vi "WindTunnel.vi"() -> ()   [LabVIEW 2019]
uses:
  <vilib>/platform/TimedLoop/XDataNode/XDataNode.xnode
  <vilib>/Platform/TimedLoop/XDataNode/nitl_modes.ctl
  <vilib>/Platform/TimedLoop/XDataNode/XDNodeRunTimeDep.lvlib
  <vilib>/Platform/TimedLoop/XDataNode/wakeup.ctl
  <vilib>/Platform/TimedLoop/XDataNode/timing_clust.ctl
  <resource>/objmgr/ni.dex.rc
panel:
  out "save_counter":dbl
  out "saving_now":bool
  out "save_array":dbl[][](array[numeric])
  out "Aux Pressure":dbl
  out "Pitot Pressure":dbl
  out "save_file":path
  out "file_header":string[](array[string])=["%Atmospheric Pressure [Pa]", "Atmospheric Temperature [K]", "Atmospheric Density [kg/m^3]", "Airspeed [m/s]", "Pitot Dynamic Pressure [Pa]", "Aux Dynamic Pressure [Pa]", "Scanivalve Pressure 1 [Pa]", "Scanivalve Pressure 2 [Pa]", "Scanivalve Pressure 3 [Pa]", "Scanivalve Pressure 4 [Pa]", "Scanivalve Pressure 5 [Pa]", "Scanivalve Pressure 6 [Pa]", "Scanivalve Pressure 7 [Pa]", "Scanivalve Pressure 8 [Pa]", "Scanivalve Pressure 9 [Pa]", "Scanivalve Pressure 10 [Pa]", "Scanivalve Pressure 11 [Pa]", "Scanivalve Pressure 12 [Pa]", "Scanivalve Pressure 13 [Pa]", "Scanivalve Pressure 14 [Pa]", "Scanivalve Pressure 15 [Pa]", "Scanivalve Pressure 16 [Pa]", "Angle of Attack [deg]", "Sting Normal Force [N]", "Sting Axial Force [N]", "Sting Pitching Moment [Nm]", "ELD Probe X axis [mm]", "ELD Probe Y axis [mm]"]
  in  "Voltage Control":bool
  out "Connected\n 2":bool
  out "error out 2":errorcluster
  in  "stop 2":bool
  out "Connected":bool
  out "error out":errorcluster
  in  "Samples per Set to Save(Set before running)":dbl=20.0 caption="Samples per Set to Save" min=1.0 max=500.0 step=1.0 format="%#_13g"
  out "Control Voltage [V]":dbl=3.233886157886598
  out "Last Y Position Sent":dbl=336.2689146979012 format="%0.2f"
  out "Last X Position Sent":dbl=535.0482220636093 format="%0.2f"
  out "Sample Sets Sent to File":dbl=4.0
  out "Sampling Rate":dbl=500.0
  out "Airspeed Dynamic\n+/- 70 Pa {6895 Pa max}":dbl=106.03006103917599
  in  "stop":bool
  in  "Zero ELD Probe Location":bool
  in  "Desired Airspeed (m/s)":dbl(knob) min=0.0 max=40.0 step=0.01 scale=0.0..40.0 scale format="%.2g"
  out "Y":dbl=336.2689146979012 format="%.2f"
  out "X":dbl=535.0482220636093 format="%.2f"
  in  "Send Samples To File":bool
  out "Actual Airspeed [m/s]":dbl(knob) caption="m/s" scale=0.0..64.8 scale format="%_3g"
  in  "Tab Control":enum32{"Pressures", "Forces", "Angle of Attack"}(tab)
  out "Scanivalve Pressures":cluster{i32[], "Array":dbl[]}(graph)={[1, 2, 3, 4, 5, 6, 7, 8, 9, 10, 11, 12, 13, 14, 15, 16], "Array"=[107.2386417388916, 109.67449417114258, 112.26835975646972, 113.32290878295899, 113.25851020812988, 110.12275047302246, 110.01677665710449, 110.23803977966308, 111.38681907653809, 112.57089157104492, 115.55567054748535, 109.39623069763184, 115.34736213684081, 113.26969871520996, 112.33615150451661, 111.57799453735352]}
  out "Atm Density [kg/m^3]":dbl=0.9456665967088438 format="%.2g"
  out "Atm Pressure [Pa]":dbl=81675.50593656283 format="%.2f"
  out "Atm Temperature [K]":dbl=300.88201803705715 format="%.2g"
  in  "Zero Airspeed & Pressures":bool
  out "Pressures Chart":dynamicdata(graph)
  out "Forces Chart":dynamicdata(graph)
  in  "Zero Forces and Moment":bool
  out "Normal Force (N) {111.2 N max}":dbl=-0.11861150697340539 format="%#_5g"
  out "Axial Force (N) {44.5 N max}":dbl=0.06610776257324563 format="%#_5g"
  out "Pitching Moment (Nm) {5.6 Nm max}":dbl=-0.0053004445096350794 format="%#_5g"
  in  "AoA Switch":bool caption="Boolean"
  in  "Zero Angle":bool
  out "Angle of Attack Chart":dbl(graph)
  out "Angle of \nAttack":dbl=-0.004685357123962319 caption="deg ±20 Max" format="%.3g"
  # "AIRSPEED"
  # "ELD PRESSURE PROBE"
  # "SAMPLES"
  # "ELD Probe Location"
  # "mm"
  # "mm"
  # "Pa"
  # "Control Parameters:"
  # "Display Parameters:"
  # "Sting Balance Reading"
  # "Manual Input"
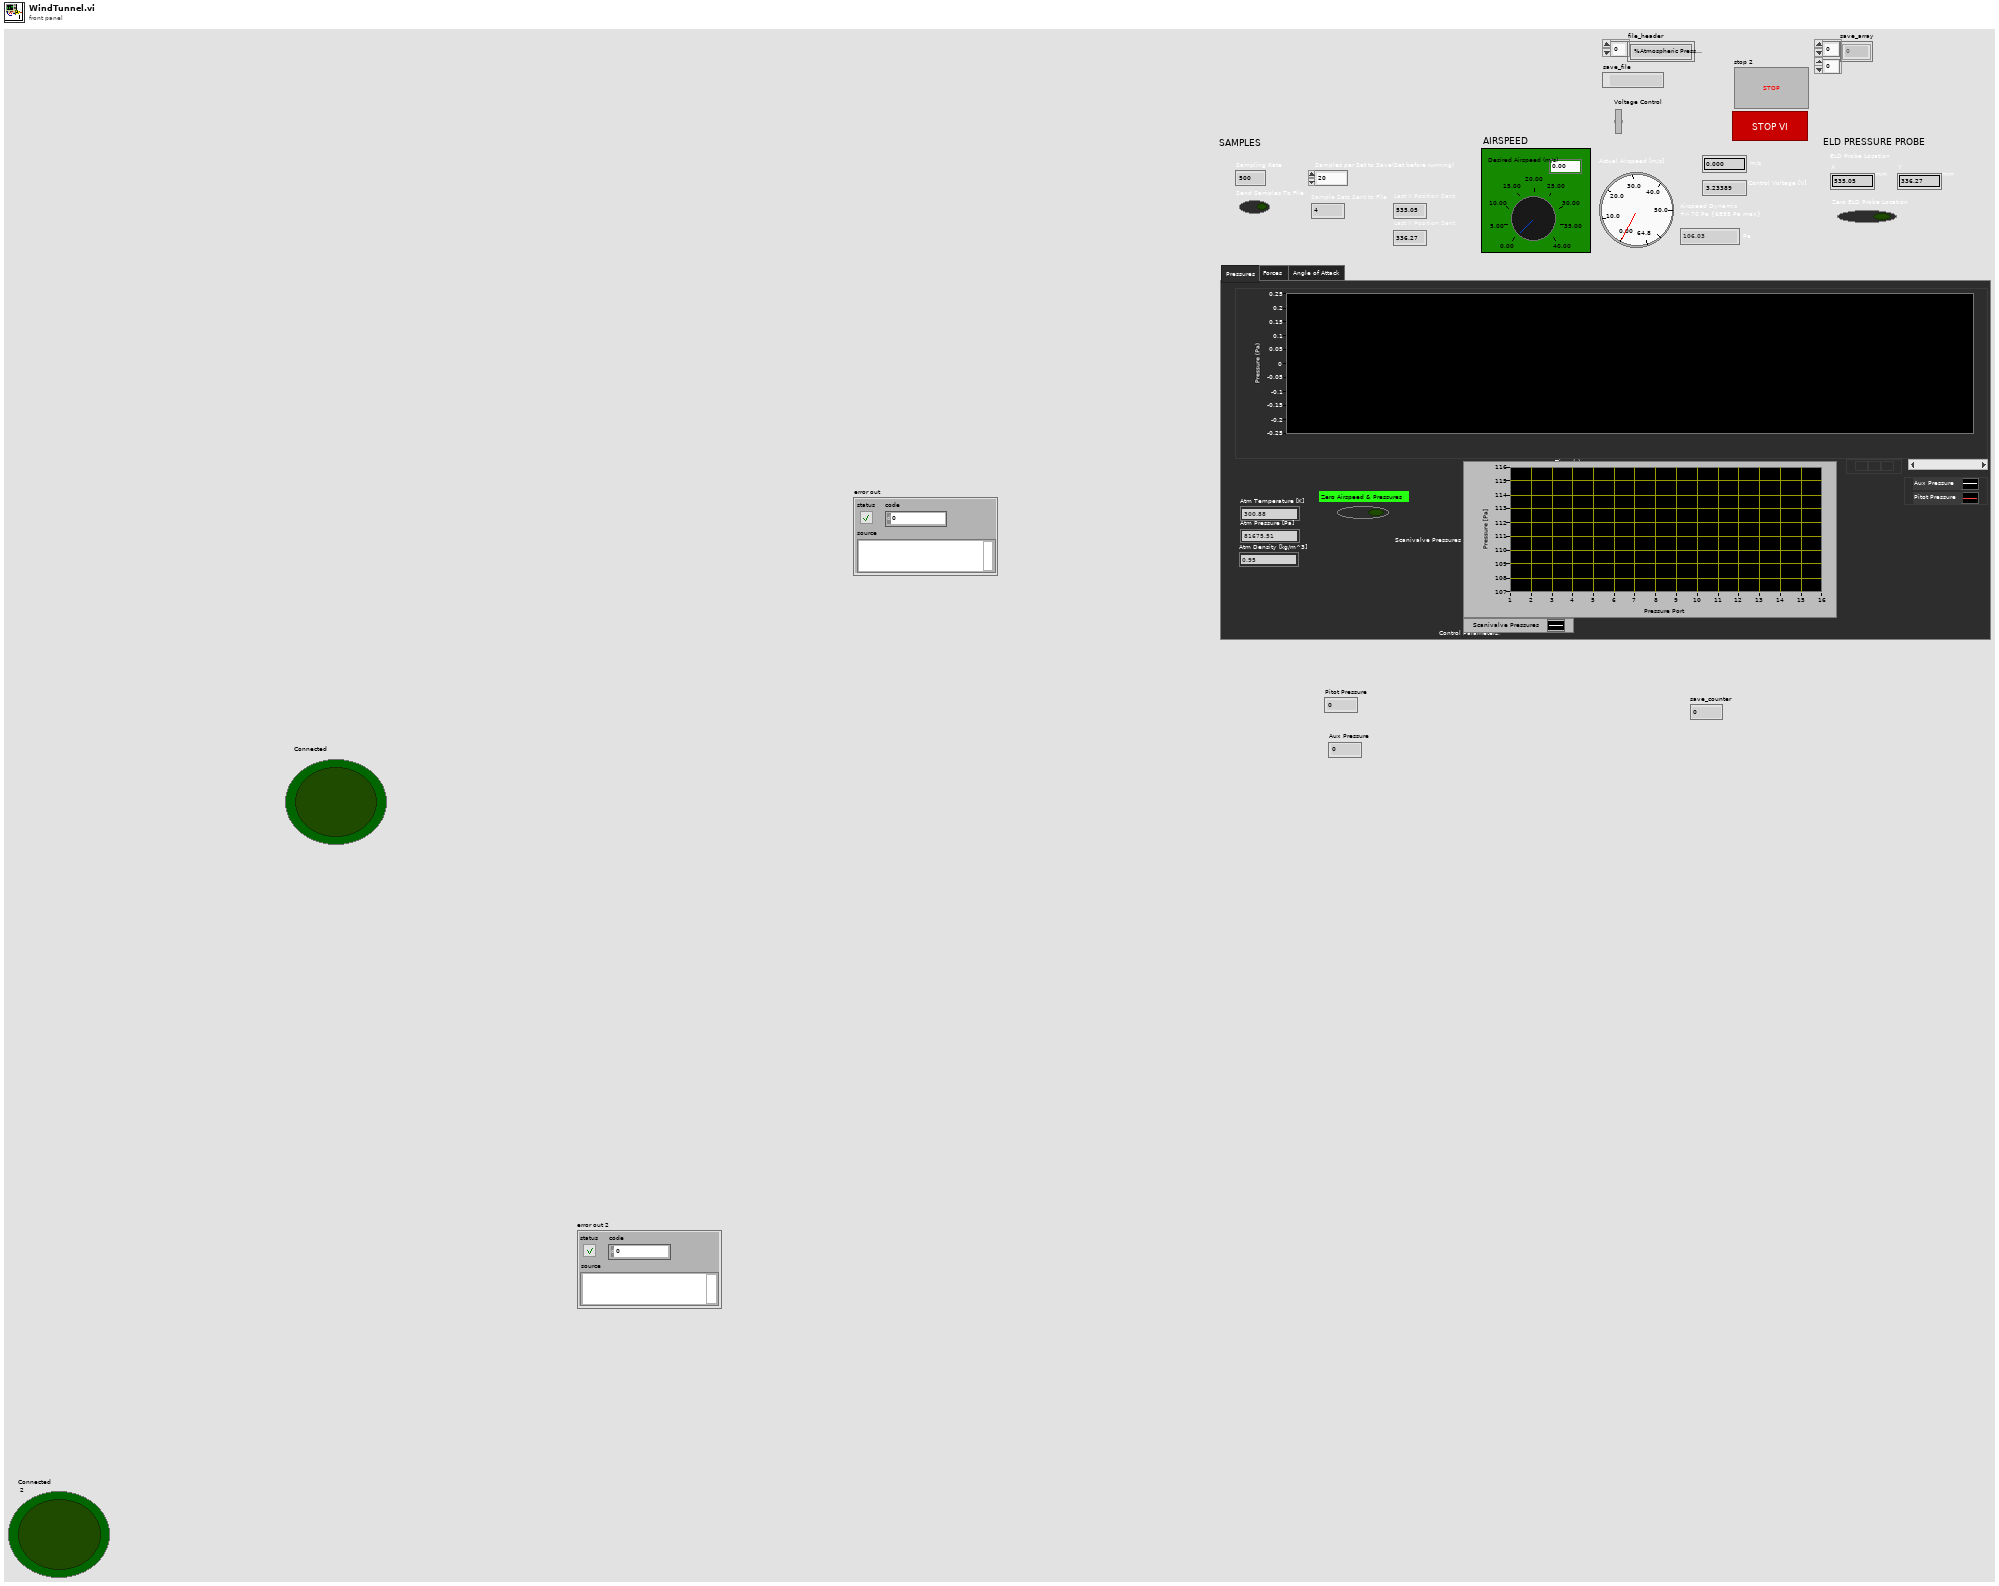
[diagram p1: front panel]
types:
  T1 = typedef "XDNodeRunTimeDep.lvlib/timing_clust.ctl" = cluster{"Expected End [f-1]":u64, "Actual End [f-1]":u64, "Finished Late? [f-1]":bool, "Expected End [i-1]":u64, "Actual End [i-1]":u64, "Finished Late? [i-1]":bool, "Expected Start [i]":u64, "Actual Start [i]":u64, "Expected Start [f]":u64, "Actual Start [f]":u64, "Source Name":string, "Structure Name":string, "Period":i64, "Deadline":i64, "Offset":i64, "Start":i64, "Priority":i32, "Timeout":i32, "Mode":T2, "Wakeup Reason":T3, "Error":errorcluster, "Source Type":string, "Secondary Source Type":string, "Global End Time":u64, "Global Start Time":u64, "Frame Duration":u64, "Iteration Duration":u64, "Assigned CPU":i32, "I/O Scan Engine Mode":u32}
  T2 = typedef "XDNodeRunTimeDep.lvlib/nitl_modes.ctl" = enum32{"No Change", "Process missed periods, maintain original phase", "Discard missed periods, maintain original phase", "Process missed periods, ignore original phase", "Discard missed periods, ignore original phase"}
  T3 = typedef "XDNodeRunTimeDep.lvlib/wakeup.ctl" = enum32{"Normal", "Aborted", "Asynchronous wakeup", "Timing source error", "Timed loop error", "Timeout"}
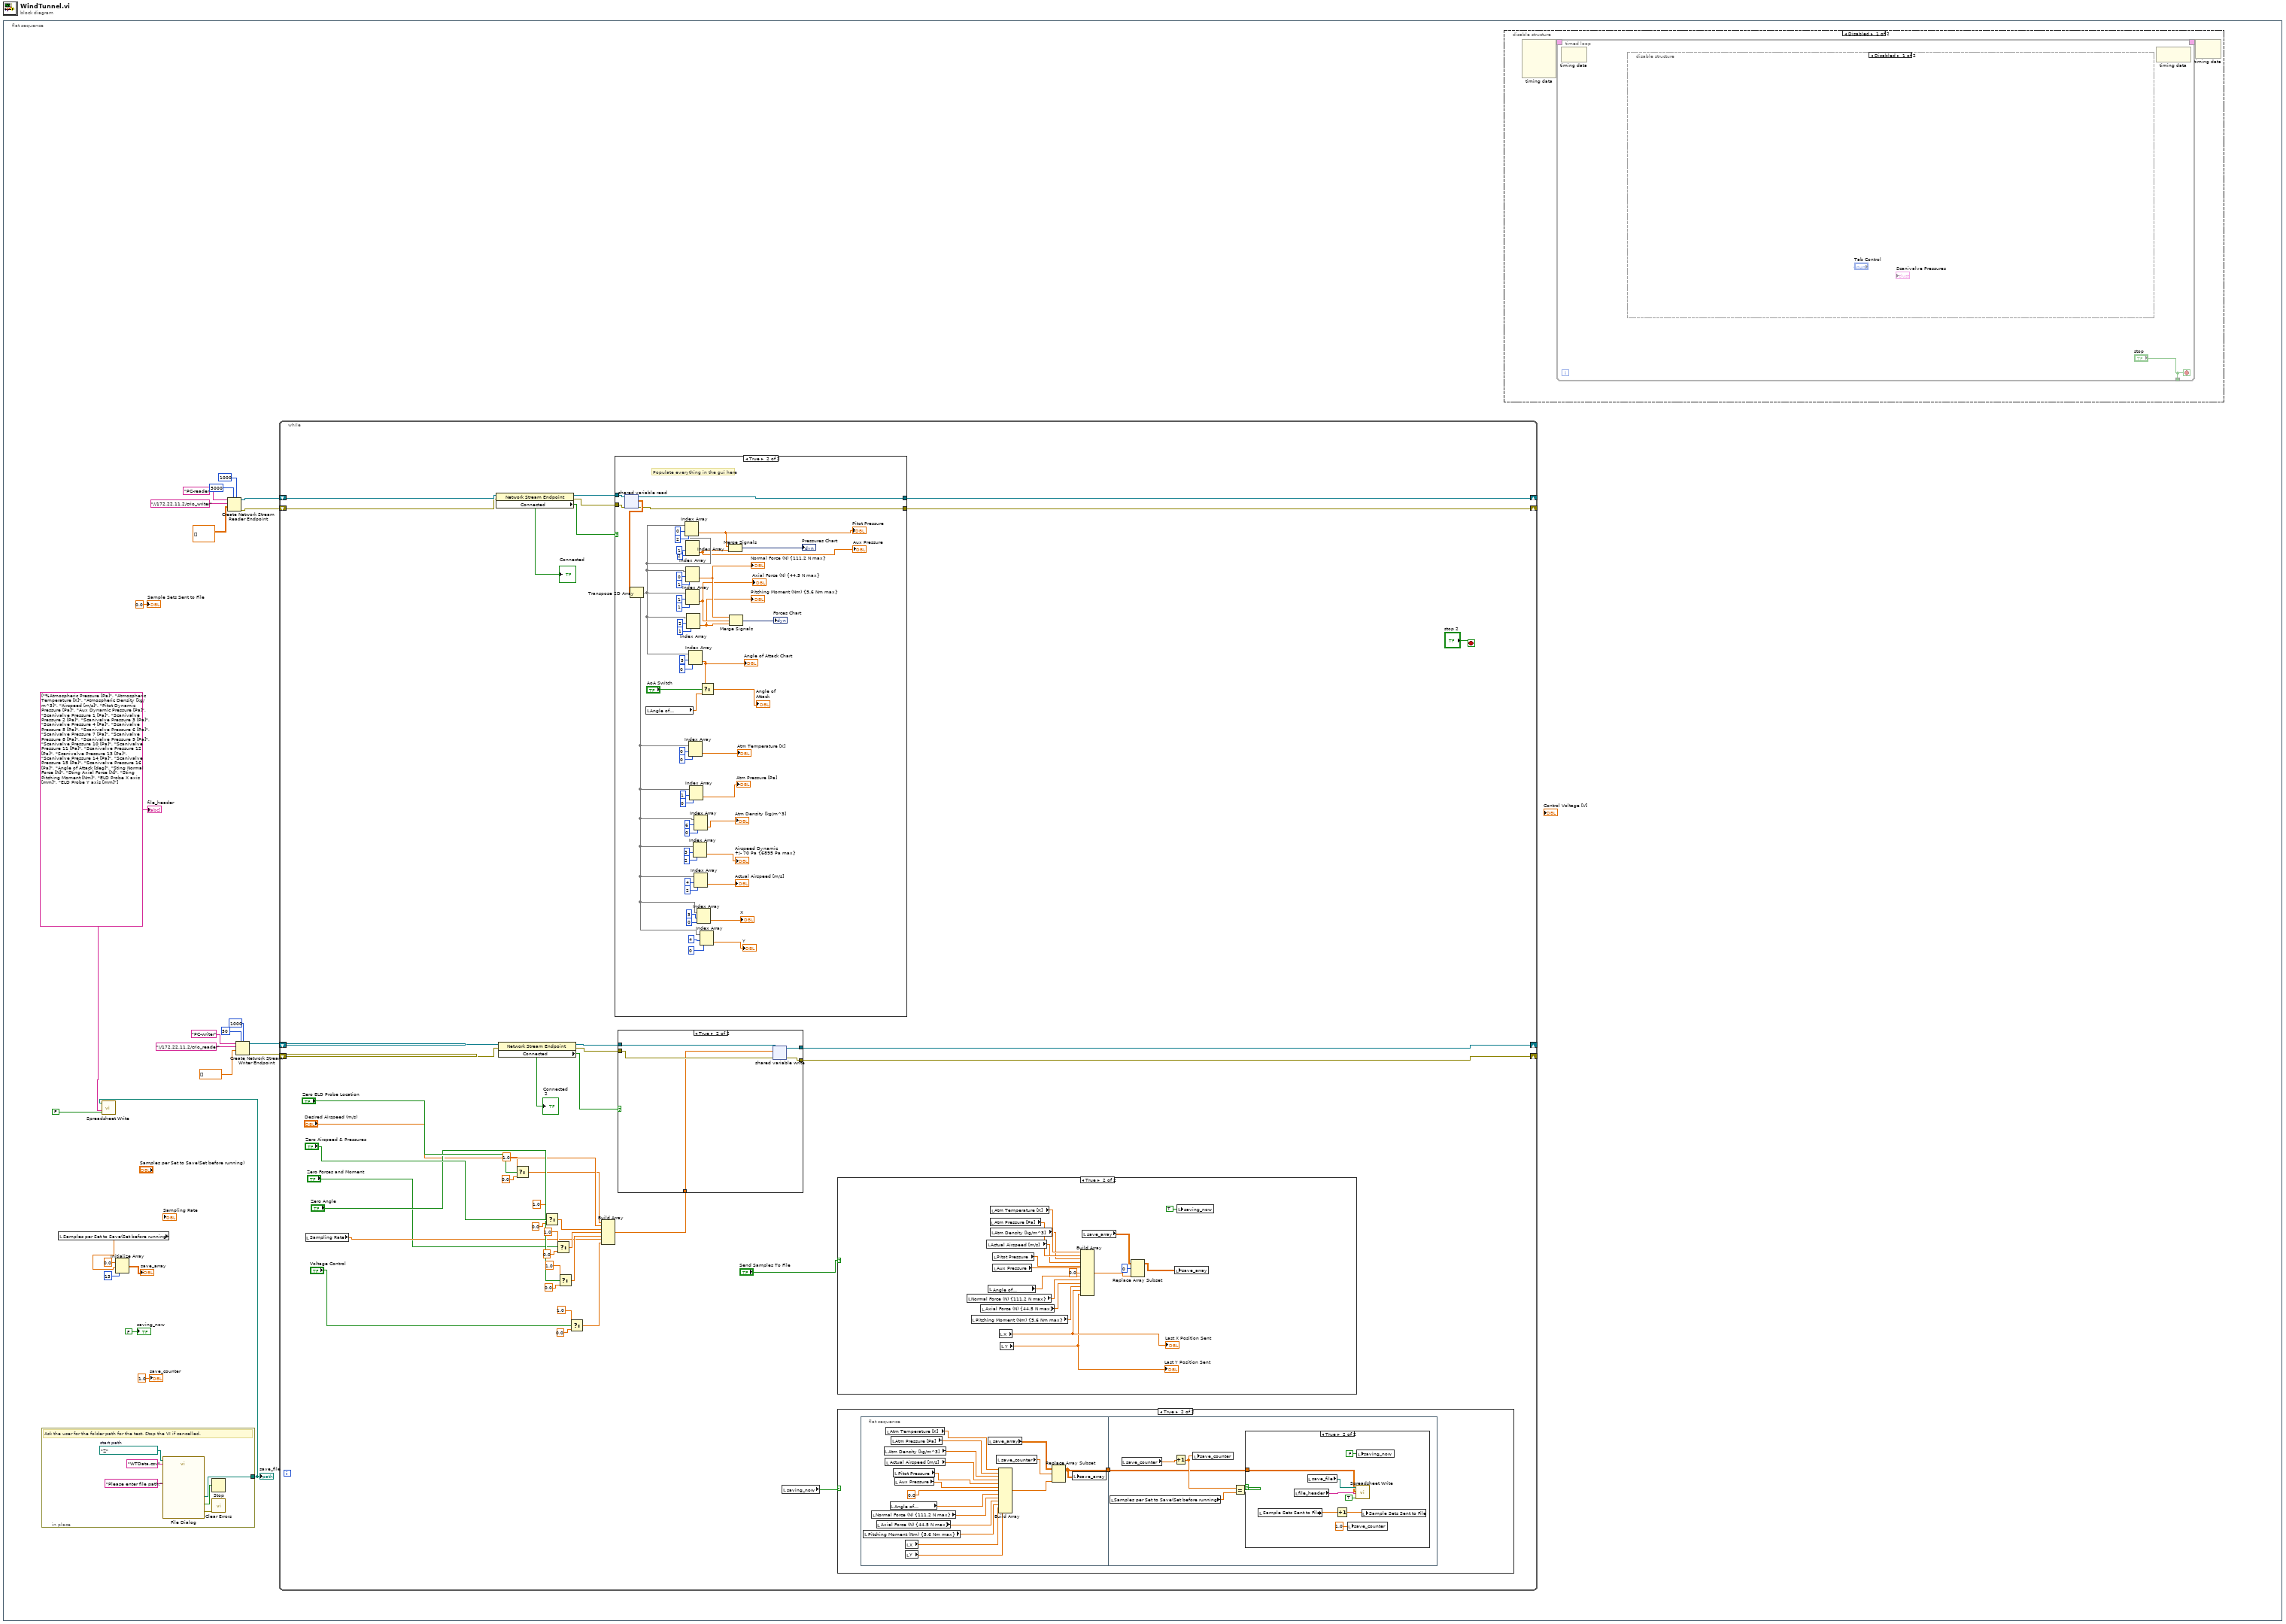
[diagram p0: block diagram]
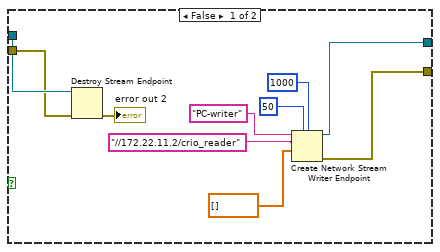
[diagram p7: hidden frame]
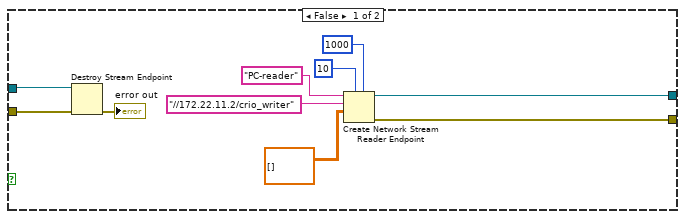
[diagram p8: hidden frame]
diagram:
  n1 = flat-sequence {
    frame #0 {
      w4 = string[] ["%Atmospheric Pressure [Pa]", "Atmospheric Temperature [K]", "Atmospheric Density [kg/m^3]", "Airspeed [m/s]", "Pitot Dynamic Pressure [Pa]", "Aux Dynamic Pressure [Pa]", "Scanivalve Pressure 1 [Pa]", "Scanivalve Pressure 2 [Pa]", "Scanivalve Pressure 3 [Pa]", "Scanivalve Pressure 4 [Pa]", "Scanivalve Pressure 5 [Pa]", "Scanivalve Pressure 6 [Pa]", "Scanivalve Pressure 7 [Pa]", "Scanivalve Pressure 8 [Pa]", "Scanivalve Pressure 9 [Pa]", "Scanivalve Pressure 10 [Pa]", "Scanivalve Pressure 11 [Pa]", "Scanivalve Pressure 12 [Pa]", "Scanivalve Pressure 13 [Pa]", "Scanivalve Pressure 14 [Pa]", "Scanivalve Pressure 15 [Pa]", "Scanivalve Pressure 16 [Pa]", "Angle of Attack [deg]", "Sting Normal Force [N]", "Sting Axial Force [N]", "Sting Pitching Moment [Nm]", "ELD Probe X axis [mm]", "ELD Probe Y axis [mm]"]
      n2 = in-place {
        in-place-border: [w26] -> w2
        w28 = path "Z:/"  # start path
        # "Ask the user for the folder path for the test. Stop the VI if cancelled."
        n3 = call "File Dialog"("start path"=w28, "prompt"="Please enter file path:" ("prompt (Create Folder)"), "default name"="WTData.csv" ("string")) -> ("selected path"=w26:path, "cancelled"=w29:bool, "error out"=w25:errorcluster)  [unwired: 9 in, 1 out]
        n4 = Stop(stop? (T)=w29) -> ()
        n5 = call <vilib>:"Clear Errors.vi"("error in (no error)"=w25) -> ()  [unwired: 5 in, 2 out]
      }
      "save_file" <- w2
      n6 = local read "Samples per Set to Save(Set before running)"() -> (w5:dbl)
      n7 = call "Spreadsheet Write.vi"("append to file? (new file:F)"=FALSE, "Header Strings"=w4, "file path (dialog if empty)"=w2) -> ()  [unwired: 4 in, 2 out]
      n8 = Initialize Array(0.0 ("element"), w5, 13 ("dimension size")) -> (→"save_array":dbl[][])
      n9 = Create Network Stream Reader Endpoint(5:1000 ("timeout in ms (-1)"), 7:5000 ("reader buffer size"), 9:dbl[][] [] ("data"), 10:"//172.22.11.2/crio_writer" ("writer url"), 11:"PC-reader" ("reader name")) -> (0:w19:errorcluster, 3:w20:refnum<k21>)  [unwired: 2 in]
      n10 = Create Network Stream Writer Endpoint(5:1000 ("timeout in ms (-1)"), 7:50 ("reader buffer size"), 9:dbl[] [] ("data"), 10:"//172.22.11.2/crio_reader" ("writer url"), 11:"PC-writer" ("reader name")) -> (0:w11:errorcluster, 3:w12:refnum<k21>)  [unwired: 2 in]
      n11 = while {
        shift-right: [w72] -> _
        shift-left: w20 -> [w77]
        shift-right: [w71] -> _
        shift-left: w19 -> [w73]
        shift-right: [w64] -> _
        shift-left: w12 -> [w66]
        shift-right: [w63] -> _
        shift-left: w11 -> [w65]
        stop <- "stop 2" stop-if-true
        n12 = local read "Sampling Rate"() -> (w45:dbl)
        n13 = property class="Network Stream Endpoint"(reference=w77, error in=w73) -> (reference out=w76:refnum<k21>, error out=w74:errorcluster, "Connected"=w75:bool)
        "Connected" <- w75
        n14 = property class="Network Stream Endpoint"(reference=w66, error in=w65) -> (reference out=w67:refnum<k21>, error out=w69:errorcluster, "Connected"=w68:bool)
        "Connected\n 2" <- w68
        n15 = Select(t=1.0, s="Zero ELD Probe Location", f=0.0) -> (s? t:f=w49:dbl)
        n16 = Select(t=1.0, s="Zero Airspeed & Pressures", f=0.0) -> (s? t:f=w48:dbl)
        n17 = Select(t=1.0, s="Zero Forces and Moment", f=0.0) -> (s? t:f=w47:dbl)
        n18 = Select(t=1.0, s="Zero Angle", f=0.0) -> (s? t:f=w46:dbl)
        n19 = Select(t=1.0, s="Voltage Control", f=0.0) -> (s? t:f=w40:dbl)
        n20 = Build Array(w49, "Desired Airspeed (m/s)", w48, w47, w46, w45, w40) -> (w58:dbl[])
        n21 = case shown="True" w75 {
          tunnel: w76 -> [w151 w201]
          tunnel: w74 -> [w150 w198]
          tunnel: [w144 w200] -> w72
          tunnel: [w143 w197] -> w71
          frame False {
            n22 = Destroy Stream Endpoint(8:w150, 11:w151) -> (0:→"error out":errorcluster)
            n23 = Create Network Stream Reader Endpoint(5:1000 ("timeout in ms (-1)"), 7:10 ("reader buffer size"), 9:dbl[][] [] ("data"), 10:"//172.22.11.2/crio_writer" ("writer url"), 11:"PC-reader" ("reader name")) -> (0:w143:errorcluster, 3:w144:refnum<k21>)  [unwired: 2 in]
          }
          frame True {
            # "Populate everything in the gui here"
            n24 = shared-variable-read(w201, w198) -> (w200:refnum<k21>, w197:errorcluster, w199:dbl[][])  [unwired: 1 in, 1 out]
            n25 = Transpose 2D Array(2D array=w199) -> (transposed array=w154:dbl[][])
            n26 = local read "Angle of \nAttack"() -> (w179:dbl)
            n27 = Index Array(array=w154, index (row)=0, index (col)=2) -> (element=w153:dbl)
            "Pitot Pressure" <- w153
            n28 = Index Array(array=w154, index (row)=1, index (col)=2) -> (element=w152:dbl)
            "Aux Pressure" <- w152
            n29 = Index Array(array=w154, index (row)=0, index (col)=1) -> (element=w172:dbl)
            "Normal Force (N) {111.2 N max}" <- w172
            n30 = Index Array(array=w154, index (row)=1, index (col)=1) -> (element=w171:dbl)
            "Axial Force (N) {44.5 N max}" <- w171
            n31 = Index Array(array=w154, index (row)=2, index (col)=1) -> (element=w170:dbl)
            "Pitching Moment (Nm) {5.6 Nm max}" <- w170
            n32 = Index Array(array=w154, index (row)=0, index (col)=0) -> (element=→"Atm Temperature [K]":dbl)
            n33 = Index Array(array=w154, index (row)=5, index (col)=0) -> (element=w181:dbl)
            "Angle of Attack Chart" <- w181
            n34 = Index Array(array=w154, index (row)=1, index (col)=0) -> (element=→"Atm Pressure [Pa]":dbl)
            n35 = Index Array(array=w154, index (row)=3, index (col)=2) -> (element=→"Airspeed Dynamic\n+/- 70 Pa {6895 Pa max}":dbl)
            n36 = Index Array(array=w154, index (row)=6, index (col)=0) -> (element=→"Atm Density [kg/m^3]":dbl)
            n37 = Index Array(array=w154, index (row)=4, index (col)=2) -> (element=→"Actual Airspeed [m/s]":dbl)
            n38 = Index Array(array=w154, index (row)=3, index (col)=0) -> (element=→"X":dbl)
            n39 = Index Array(array=w154, index (row)=4, index (col)=0) -> (element=→"Y":dbl)
            n40 = Select(t=w181, s="AoA Switch", f=w179) -> (s? t:f=→"Angle of \nAttack":dbl)
            n41 = Merge Signals(w153, w152) -> (→"Pressures Chart":dynamicdata)
            n42 = Merge Signals(w172, w171, w170) -> (→"Forces Chart":dynamicdata)
          }
        }
        n43 = case shown="True" w68 {
          tunnel: w67 -> [w136 w139]
          tunnel: w69 -> [w135 w141]
          tunnel: [w128 w138] -> w64
          tunnel: [w127 w140] -> w63
          tunnel: w58 -> [_ w137]
          frame False {
            n44 = Destroy Stream Endpoint(8:w135, 11:w136) -> (0:→"error out 2":errorcluster)
            n45 = Create Network Stream Writer Endpoint(5:1000 ("timeout in ms (-1)"), 7:50 ("reader buffer size"), 9:dbl[] [] ("data"), 10:"//172.22.11.2/crio_reader" ("writer url"), 11:"PC-writer" ("reader name")) -> (0:w127:errorcluster, 3:w128:refnum<k21>)  [unwired: 2 in]
          }
          frame True {
            n46 = shared-variable-write(w139, w141, w137) -> (w138:refnum<k21>, w140:errorcluster)  [unwired: 1 in, 1 out]
          }
        }
        n47 = local read "saving_now"() -> (w38:bool)
        n48 = case shown="True" w38 {
          frame False {
          }
          frame True {
            n49 = flat-sequence {
              tunnel: [w80] -> w78
              tunnel: w78 -> [w96]
              frame #0 {
                n50 = local read "Pitching Moment (Nm) {5.6 Nm max}"() -> (w86:dbl)
                n51 = local read "Normal Force (N) {111.2 N max}"() -> (w88:dbl)
                n52 = local read "Axial Force (N) {44.5 N max}"() -> (w87:dbl)
                n53 = local read "Atm Density [kg/m^3]"() -> (w93:dbl)
                n54 = local read "Actual Airspeed [m/s]"() -> (w92:dbl)
                n55 = local read "Atm Temperature [K]"() -> (w95:dbl)
                n56 = local read "Angle of \nAttack"() -> (w89:dbl)
                n57 = local read "Atm Pressure [Pa]"() -> (w94:dbl)
                n58 = local read "Pitot Pressure"() -> (w91:dbl)
                n59 = local read "Aux Pressure"() -> (w90:dbl)
                n60 = local read "X"() -> (w85:dbl)
                n61 = local read "Y"() -> (w84:dbl)
                n62 = local read "save_array"() -> (w82:dbl[][])
                n63 = local read "save_counter"() -> (w79:dbl)
                n64 = Build Array(w95, w94, w93, w92, w91, w90, 0.0 ("element"), w89, w88, w87, w86, w85, w84) -> (w81:dbl[])
                n65 = Replace Array Subset(array=w82, new element=w81, index (row)=w79) -> (w80:dbl[][])  [unwired: 1 in]
                n66 = local write "save_array"(w80) -> ()
              }
              frame #1 {
                n67 = local read "Samples per Set to Save(Set before running)"() -> (w100:dbl)
                n68 = local read "save_counter"() -> (w98:dbl)
                n69 = Increment(x=w98) -> (x+1=w99:dbl)
                n70 = local write "save_counter"(w99) -> ()
                n71 = Equal?(x=w99, y=w100) -> (x = y?=w97:bool)
                n72 = case shown="True" w97 {
                  tunnel: w96 -> [_ w105]
                  frame False {
                  }
                  frame True {
                    n73 = local read "Sample Sets Sent to File"() -> (w102:dbl)
                    n74 = local read "file_header"() -> (w107:string[])
                    n75 = local read "save_file"() -> (w108:path)
                    n76 = Increment(x=w102) -> (x+1=w101:dbl)
                    n77 = local write "save_counter"(1.0 ("save_counter")) -> ()
                    n78 = call "Spreadsheet Write.vi"("append to file? (new file:F)"=TRUE, "Header Strings"=w107, "2D data"=w105, "file path (dialog if empty)"=w108) -> ()  [unwired: 3 in, 2 out]
                    n79 = local write "saving_now"(FALSE ("saving_now")) -> ()
                    n80 = local write "Sample Sets Sent to File"(w101) -> ()
                  }
                }
              }
            }
          }
        }
        n81 = case shown="True" "Send Samples To File" {
          frame False {
          }
          frame True {
            n82 = local read "Normal Force (N) {111.2 N max}"() -> (w119:dbl)
            n83 = local read "Pitching Moment (Nm) {5.6 Nm max}"() -> (w117:dbl)
            n84 = local read "Axial Force (N) {44.5 N max}"() -> (w118:dbl)
            n85 = local read "Actual Airspeed [m/s]"() -> (w123:dbl)
            n86 = local read "Angle of \nAttack"() -> (w120:dbl)
            n87 = local read "Atm Pressure [Pa]"() -> (w125:dbl)
            n88 = local read "Atm Temperature [K]"() -> (w126:dbl)
            n89 = local read "Atm Density [kg/m^3]"() -> (w124:dbl)
            n90 = local read "Pitot Pressure"() -> (w122:dbl)
            n91 = local read "Aux Pressure"() -> (w121:dbl)
            n92 = local read "X"() -> (w110:dbl)
            "Last X Position Sent" <- w110
            n93 = local read "Y"() -> (w109:dbl)
            "Last Y Position Sent" <- w109
            n94 = Build Array(w126, w125, w124, w123, w122, w121, 0.0 ("element"), w120, w119, w118, w117, w110, w109) -> (w114:dbl[])
            n95 = local read "save_array"() -> (w112:dbl[][])
            n96 = Replace Array Subset(array=w112, new element=w114, index (row)=0 ("index")) -> (w111:dbl[][])  [unwired: 1 in]
            n97 = local write "save_array"(w111) -> ()
            n98 = local write "saving_now"(TRUE ("saving_now")) -> ()
          }
        }
      }
      n99 = disable-structure shown="Disabled" {
        frame Disabled {
          n100 = node-c288() -> (w32:T1)  [unwired: 4 in]
          n101 = timed-loop {
            timing: w32 -> [_]
            timing-out: [_] -> w31
            tunnel: ["stop"] -> _
            stop <- "stop" stop-if-true
            n102 = node-c288() -> ()  [unwired: 1 in, 1 out]
            n103 = disable-structure shown="Disabled" {
              frame Disabled {
              }
              frame Enabled {
              }
            }
            n104 = node-c288() -> ()  [unwired: 1 in, 1 out]
          }
          n105 = node-c288(w31) -> ()  [unwired: 1 out]
        }
        frame Enabled {
        }
      }
      "file_header" <- w4
      "saving_now" <- FALSE ("saving_now")
      "save_counter" <- 1.0 ("save_counter")
      "Sample Sets Sent to File" <- 0.0 ("Sample Sets Sent to File")
    }
  }
